vi "add set current(SubVI).vi"() -> (1 "ok or cancel":bool=TRUE, 2 "连接的字符串":string)   [LabVIEW 2019, in "SubVI.lvlib"]
uses:
  SubVI.lvlib
panel:
  in  "Frequency(Hz)":dbl=13.0 format="%#_13g"
  in  "Current Amplitude":dbl
  in  "cancel":bool
  in  "ok":bool
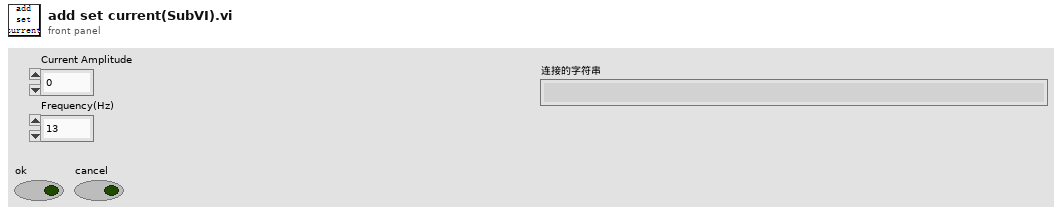
[diagram p1: front panel]
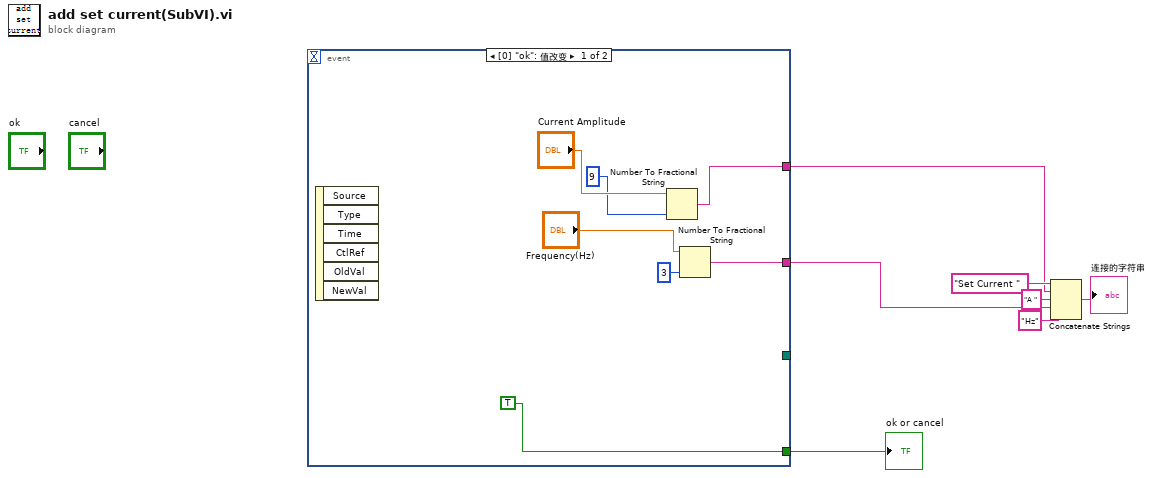
[diagram p0: block diagram]
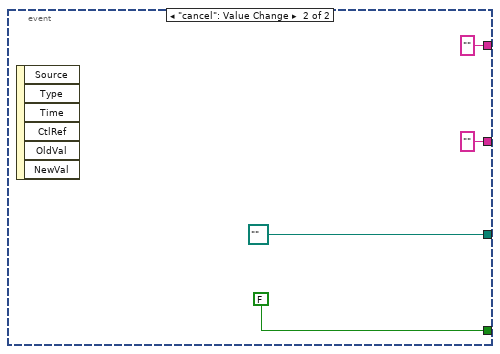
[diagram p2: hidden frame]
diagram:
  n1 = event shown="[0] \"ok\": 值改变" {
    selector: _ -> [_ _]
    dyn-events: _ -> [_ _]
    timeout: _ -> [_ _]
    tunnel: [_ path "" ("path")] -> _
    tunnel: [TRUE FALSE] -> w5
    tunnel: [w11 ""] -> w3
    tunnel: [w8 ""] -> w1
    event "ok": Value Change {
      n2 = event-data() -> ()  [unwired: 1 in, 6 out]
      n3 = Number To Fractional String(number="Current Amplitude", precision (6)=i16 9 ("精度(6)")) -> (F-format string=w11:string)  [unwired: 2 in]
      n4 = Number To Fractional String(number="Frequency(Hz)", precision (6)=i16 3 ("精度(6)")) -> (F-format string=w8:string)  [unwired: 2 in]
    }
    event "cancel": Value Change {
      n5 = event-data() -> ()  [unwired: 1 in, 6 out]
    }
  }
  "ok or cancel" <- w5
  n6 = Concatenate Strings("Set Current " ("字符串"), w3, "A " ("字符串"), w1, "Hz" ("字符串")) -> (→"连接的字符串":string)
